vi "daqStreamReaderSubVi.vi"(0 "Refnum in":refnum<k21>, 1 "OPC UA client refnum in":T1, 5 "new file path (Not A Path if cancelled)":path, 7 "OPC UA Connection Status":bool, 11 "error in (no error)":errorcluster) -> (4 "Refnum out":refnum<k21>, 6 "DAQ?":bool, 8 "Available Elements for Reading":i32, 10 "Number of Disconnections":u32, 15 "error out 3":errorcluster)   [LabVIEW 2017]
uses:
  <vilib>/OPCUA/controls/OPC UA Client Refnum.ctl
  <vilib>/Utility/file.llb/Write Delimited Spreadsheet (DBL).vi
  <resource>/objmgr/ni.dex.rc
panel:
  out "error out":errorcluster
  out "error out":errorcluster
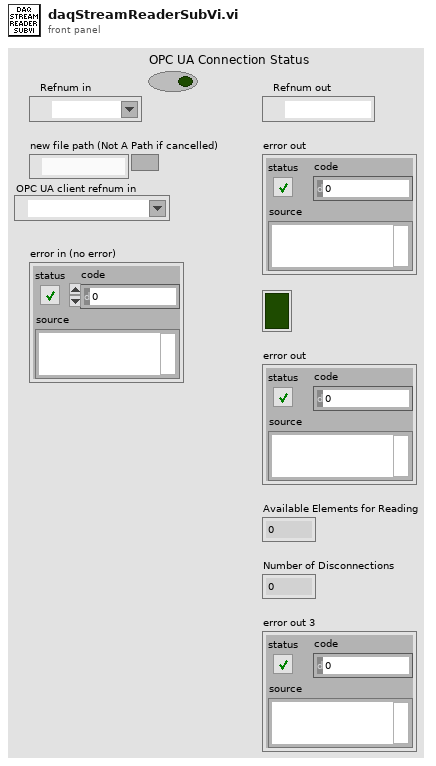
[diagram p1: front panel]
types:
  T1 = typedef "OPC UA Client Refnum.ctl" = refnum<k21>
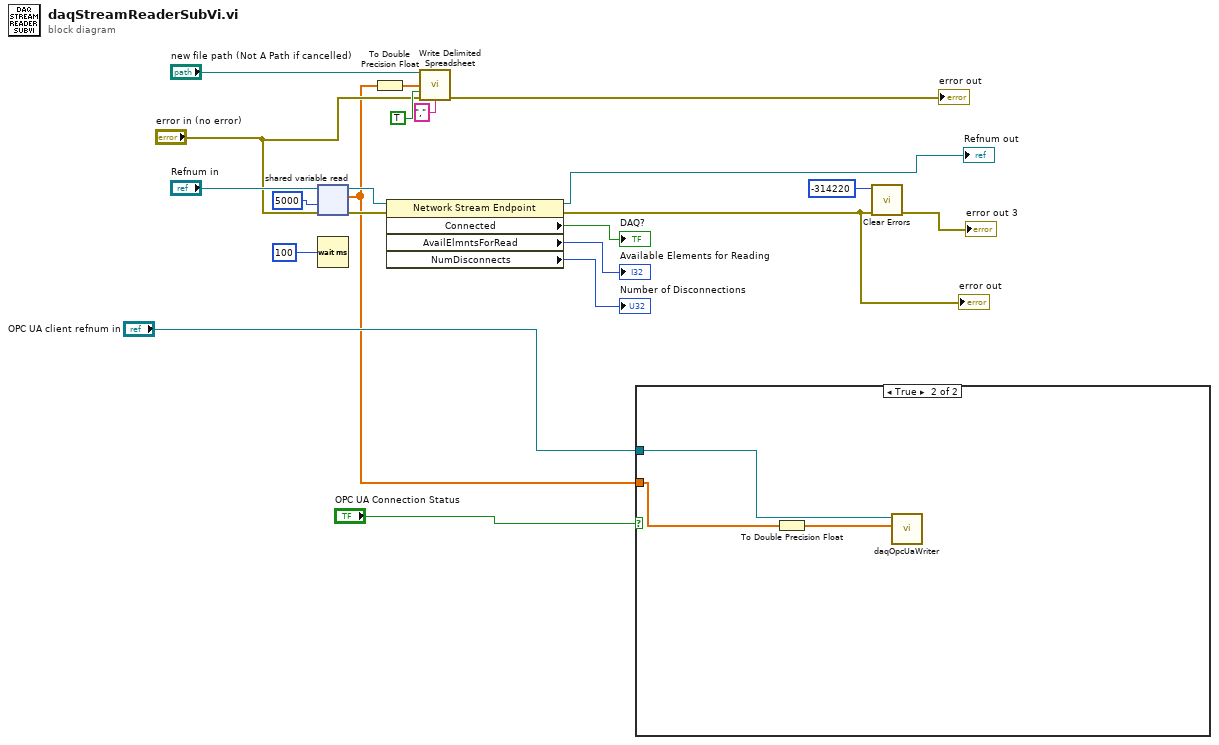
[diagram p0: block diagram]
diagram:
  n1 = shared-variable-read("Refnum in", "error in (no error)", 5000 ("timeout ms (-1)")) -> (w9:refnum<k21>, w10:errorcluster, w1:sgl[])  [unwired: 1 out]
  n2 = Wait (ms)(milliseconds to wait=u32 100) -> ()  [unwired: 1 out]
  n3 = To Double Precision Float(number=w1) -> (double precision float=w21:dbl[])
  n4 = property class="Network Stream Endpoint"(reference=w9, error in=w10) -> (reference out=→"Refnum out":refnum<k21>, error out=w5:errorcluster, "Connected"=→"DAQ?":bool, "AvailElmntsForRead"=→"Available Elements for Reading":i32, "NumDisconnects"=→"Number of Disconnections":u32)
  "error out" <- w5
  n5 = call-poly <vilib>:"Write Delimited Spreadsheet.vi"("file path (dialog if empty)"="new file path (Not A Path if cancelled)", "1D data"=w21, "append to file? (new file:F)"=TRUE, "error in (no error)"="error in (no error)", "delimiter (\\t)"="," ("delimiter (\\t)")) -> ("error out"=→"error out":errorcluster)  [unwired: 9 in, 1 out]
  n6 = case shown="True" "OPC UA Connection Status" {
    tunnel: "OPC UA client refnum in" -> [_ w24]
    tunnel: w1 -> [_ w22]
    frame False {
    }
    frame True {
      n7 = To Double Precision Float(number=w22) -> (double precision float=w23:dbl[])
      n8 = call "daqOpcUaWriter.vi"("DAQ Data Stream"=w23, "OPC UA client refnum in"=w24) -> ()  [unwired: 10 in]
    }
  }
  n9 = call <vilib>:"Clear Errors.vi"("error in (no error)"=w5, "specific error code to clear (0: all)"=-314220) -> ("error out"=→"error out 3":errorcluster)  [unwired: 4 in, 1 out]
